vi "Error Range Type.vi"(10 "Codes":string) -> (2 "Type":T1)   [LabVIEW 2014]
uses:
  Controls/Shared/SEH Code Types.ctl
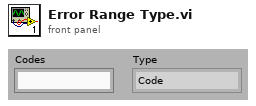
[diagram p1: front panel]
types:
  T1 = typedef "SEH Code Types.ctl" = enum16{"Code", "Range", "Category", "Invalid", "Default Action"}
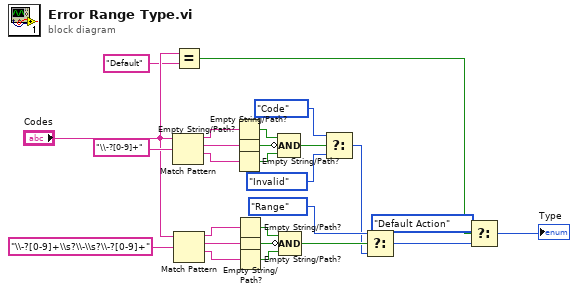
[diagram p0: block diagram]
diagram:
  n1 = Match Pattern(string="Codes", regular expression="\\-?[0-9]+") -> (before substring=w25:string, match substring=w24:string, after substring=w26:string)  [unwired: 2 out]
  n2 = Equal?(x="Codes", y="Default") -> (x = y?=w4:bool)
  n3 = Match Pattern(string="Codes", regular expression="\\-?[0-9]+\\s?\\-\\s?\\-?[0-9]+") -> (before substring=w11:string, match substring=w12:string, after substring=w10:string)  [unwired: 2 out]
  n4 = Empty String/Path?(string/path=w25) -> (empty?=w23:bool)
  n5 = Empty String/Path?(string/path=w24) -> (empty?=w22:bool)
  n6 = Empty String/Path?(string/path=w26) -> (empty?=w21:bool)
  n7 = Empty String/Path?(string/path=w11) -> (empty?=w13:bool)
  n8 = Empty String/Path?(string/path=w12) -> (empty?=w14:bool)
  n9 = Empty String/Path?(string/path=w10) -> (empty?=w15:bool)
  n10 = Compound Arithmetic op=AND(w23, invert w22, w21) -> (w20:bool)
  n11 = Compound Arithmetic op=AND(w13, invert w14, w15) -> (w16:bool)
  n12 = Select(t=SEH_Code_Types."Code", s=w20, f=SEH_Code_Types."Invalid") -> (s? t:f=w9:T1)
  n13 = Select(t=SEH_Code_Types."Range", s=w16, f=w9) -> (s? t:f=w3:T1)
  n14 = Select(t=SEH_Code_Types."Default Action", s=w4, f=w3) -> (s? t:f=→"Type":T1)
